vi "inclino._up3.vi"() -> ()   [LabVIEW 2023]
doc: "This example performs a serial port write and a serial port read. The parameters set for the serial port must match the parameters of the connected instrument or device. The VISA Configure Serial Port VI sets the configuration parameters. The front panel displays the controls used to configure the basic parameters, such as baud rate, data bits, and parity. The VI passes the VISA resource name to other VIs that perform operations on that VISA resource. The VISA Write function sends a command to the serial device and the VISA Read function returns data based on the command. The VISA Close function then closes the reference to the serial device. It is important to close the reference; otherwise, further communication through that port might not be possible."
uses:
  <vilib>/Instr/_visa.llb/VISA Configure Serial Port (Instr).vi
  Program Files (x86)/National Instruments/LabVIEW 2023/examples/Instrument IO/Serial/support/Serial - Settings.ctl
panel:
  out "Connected":bool
  out "Error Status":bool
  out "Connected":bool
  out "Error status":bool
  in  "Tab Control":enum32{"Page 1", "Page 2"}(tab)
  out "XY Graph":cluster{dbl[], dbl[]}(graph)
  out "VISA resource name out 2":refnum<visa-resource-name>
  out "VISA resource name out":refnum<visa-resource-name>
  out "?":dbl[][](array[numeric])
  in  "Referance Angle":string="!157:SOUT?\n"
  in  "Angle":string="!157:SOUT?\n"
  in  "Stop":bool
  out "?":dbl(knob) scale=-60.0..60.0
  out "?":dbl(knob) scale=-60.0..60.0
  out "Angle":dbl
  in  "Serial Settings 2":T1={"baud rate"=9600, "data bits"=8, "parity"=enum."None", "stop bits"=10, "flow control"=0} {"flow control" items=["None"=0, "XON/XOFF"=1, "RTS/CTS"=2, "DTR/DSR"=4]; "stop bits" items=["1.0"=10, "1.5"=15, "2.0"=20]; "data bits" min=5 max=8 step=1; "baud rate" items=["75"=75, "110"=110, "134"=134, "150"=150, "300"=300, "600"=600, "1200"=1200, "1800"=1800, "2400"=2400, "4800"=4800, "7200"=7200, "9600"=9600, "14400"=14400, "19200"=19200, "28800"=28800, "38400"=38400, "56000"=56000, "57600"=57600, "115200"=115200, "128000"=128000, "230400"=230400]}
  in  "PORT":refnum<visa-resource-name>="COM1"
  out "error out 2":errorcluster
  out "error out":errorcluster
  out "Referance  Angle":dbl
  in  "Serial Settings":T1={"baud rate"=9600, "data bits"=8, "parity"=enum."None", "stop bits"=10, "flow control"=0} {"flow control" items=["None"=0, "XON/XOFF"=1, "RTS/CTS"=2, "DTR/DSR"=4]; "stop bits" items=["1.0"=10, "1.5"=15, "2.0"=20]; "data bits" min=5 max=8 step=1; "baud rate" items=["75"=75, "110"=110, "134"=134, "150"=150, "300"=300, "600"=600, "1200"=1200, "1800"=1800, "2400"=2400, "4800"=4800, "7200"=7200, "9600"=9600, "14400"=14400, "19200"=19200, "28800"=28800, "38400"=38400, "56000"=56000, "57600"=57600, "115200"=115200, "128000"=128000, "230400"=230400]}
  in  "PORT":refnum<visa-resource-name>="COM1"
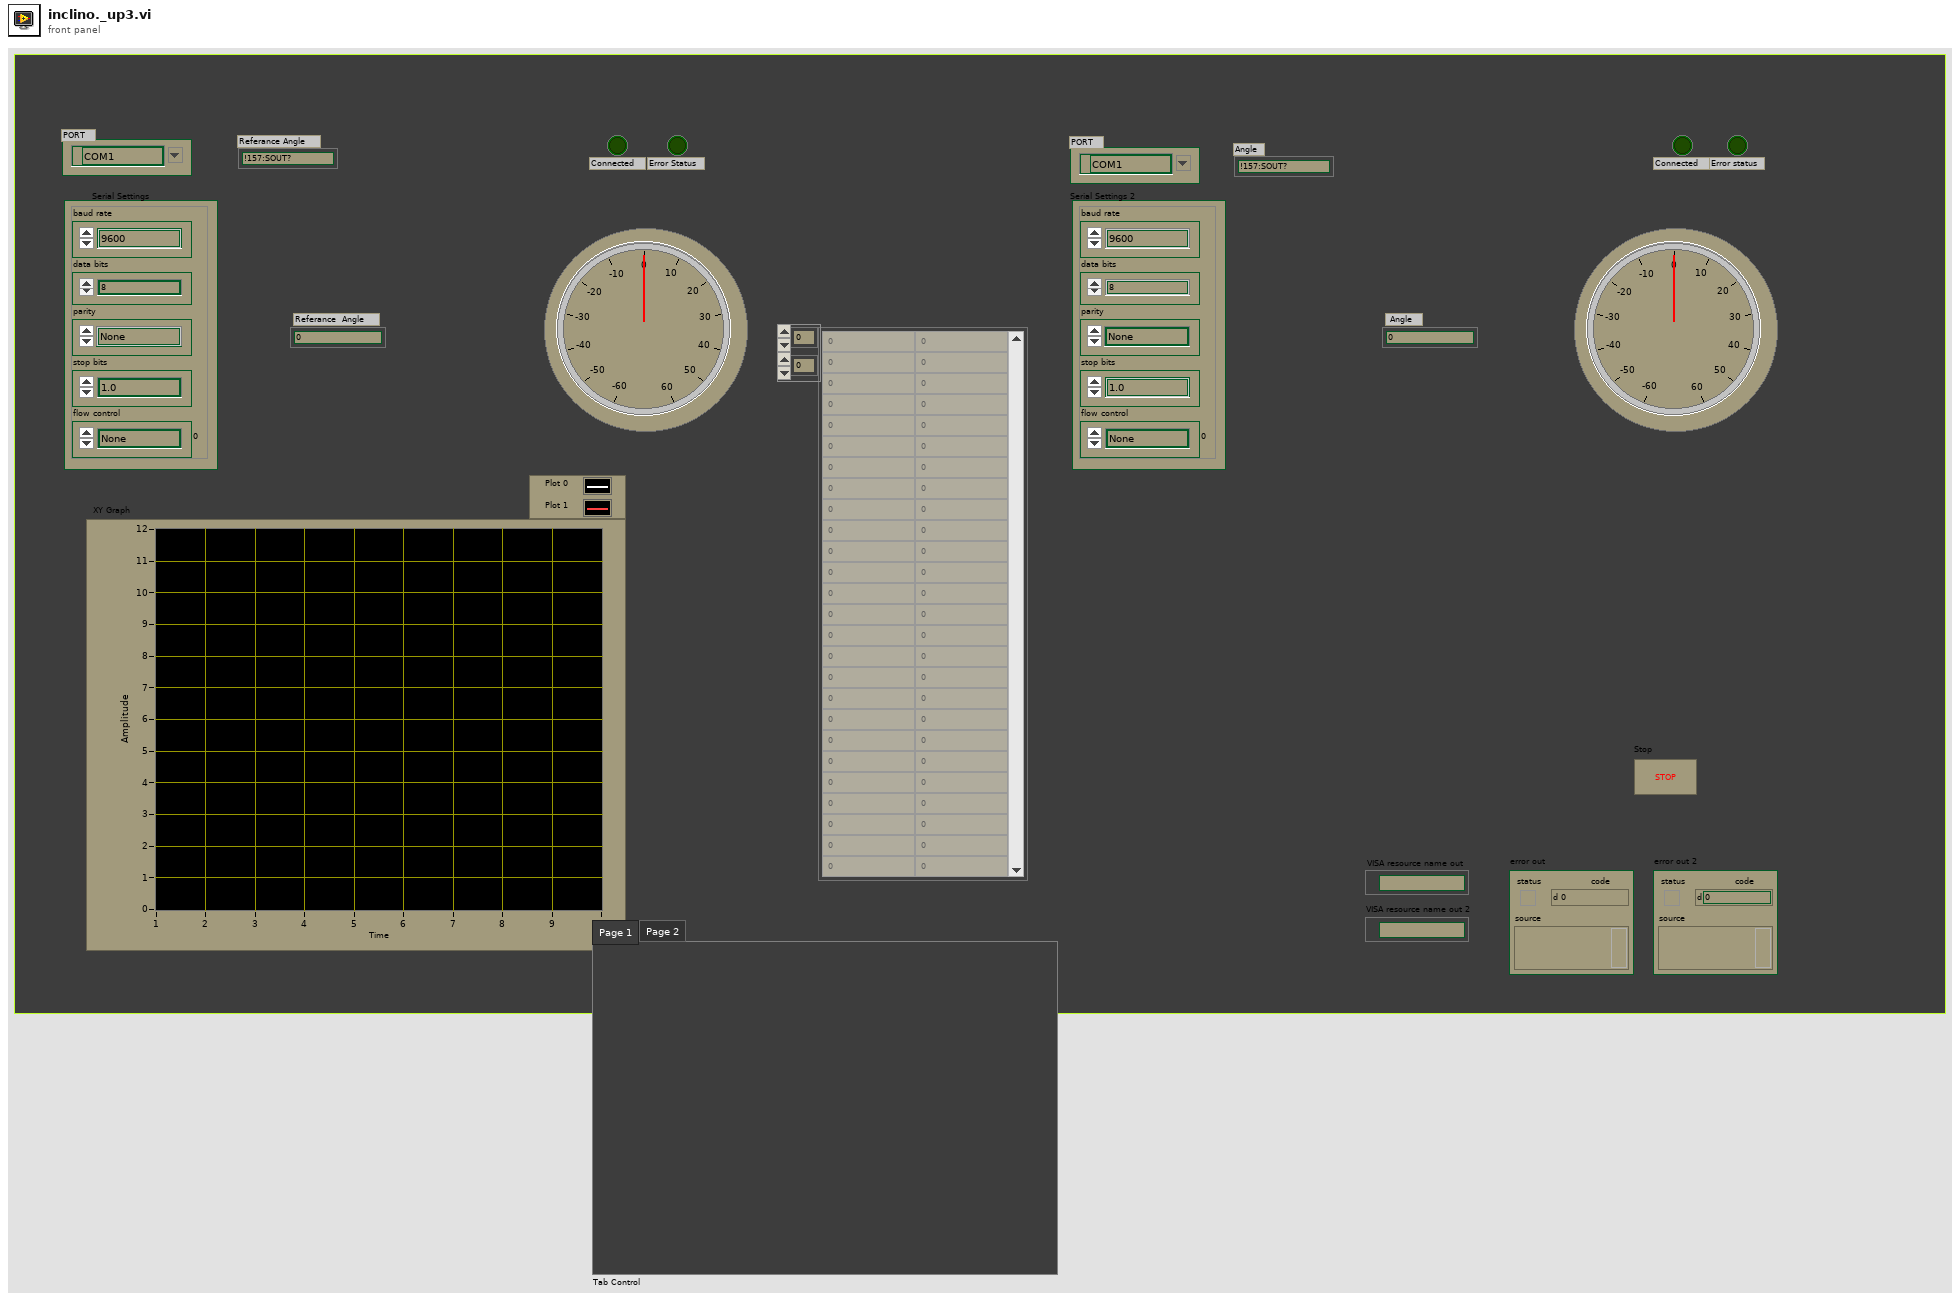
[diagram p1: front panel]
types:
  T1 = typedef "Serial - Settings.ctl" = cluster{"baud rate":u32, "data bits":u16, "parity":enum16{"None", "Odd", "Even", "Mark", "Space"}, "stop bits":u16, "flow control":u16}
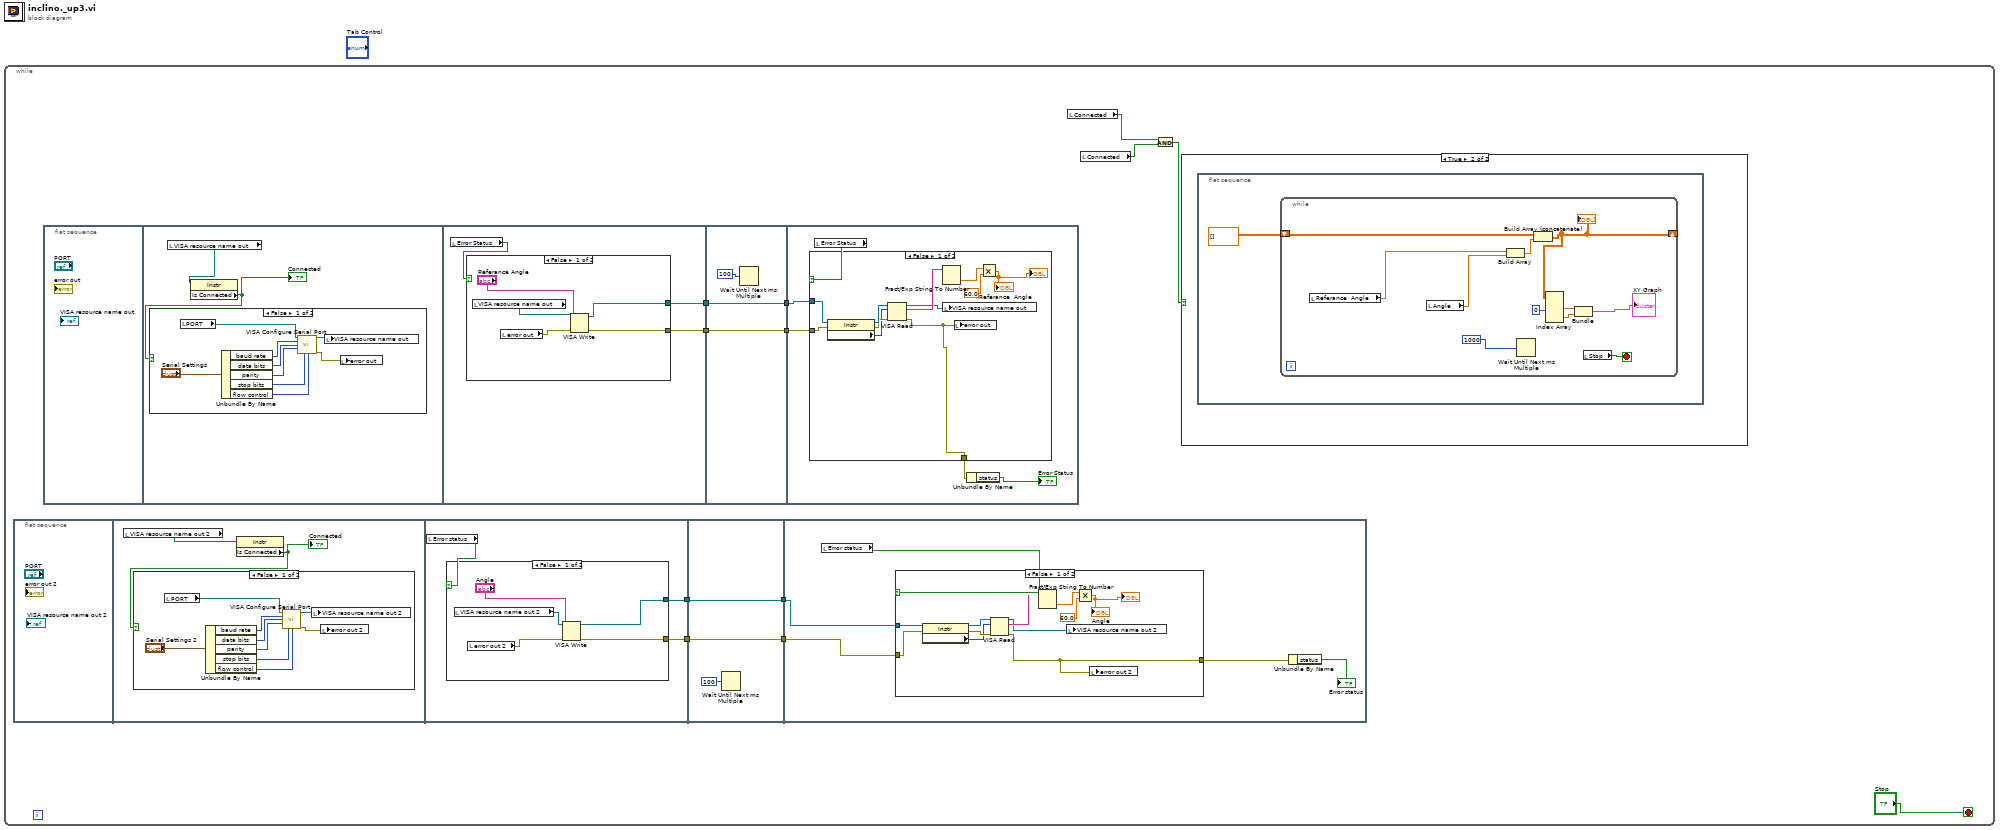
[diagram p0: block diagram]
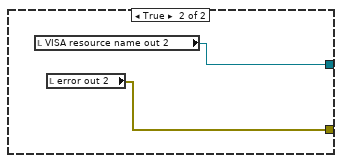
[diagram p4: hidden frame]
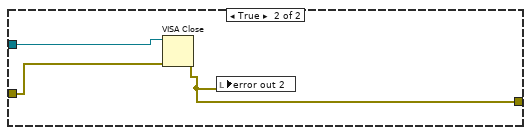
[diagram p5: hidden frame]
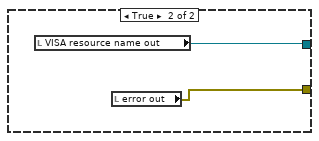
[diagram p7: hidden frame]
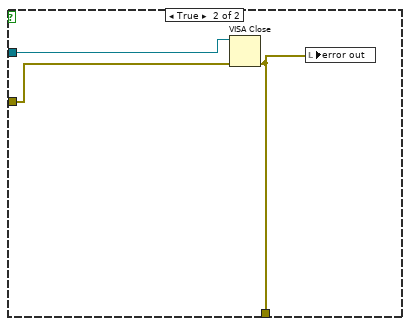
[diagram p8: hidden frame]
diagram:
  n1 = while {
    stop <- "Stop" stop-if-true
    n2 = flat-sequence {
      tunnel: [w38] -> w6
      tunnel: [w37] -> w4
      tunnel: [w47] -> w7
      tunnel: w6 -> [w47]
      tunnel: [w46] -> w5
      tunnel: w4 -> [w46]
      tunnel: w5 -> [w50]
      tunnel: w7 -> [w51]
      frame #0 {
      }
      frame #1 {
        n3 = local read "VISA resource name out 2"() -> (w26:refnum<visa-resource-name>)
        n4 = property class="Instr"(reference=w26) -> ("Is Connected"=w25:bool)  [unwired: 1 in, 2 out]
        "Connected" <- w25
        n5 = case shown="False" w25 {
          frame False {
            n6 = local read "PORT"() -> (w29:refnum<visa-resource-name>)
            n7 = Unbundle By Name("Serial Settings 2") -> ("baud rate"=w30:u32, "data bits"=w31:u16, "parity"=w32:enum16{"None", "Odd", "Even", "Mark", "Space"}, "stop bits"=w33:u16, "flow control"=w34:u16)
            n8 = call-poly "VISA Configure Serial Port"("VISA resource name"=w29, "baud rate (9600)"=w30, "data bits (8)"=w31, "parity (0:none)"=w32, "stop bits (10: 1 bit)"=w33, "flow control (0:none)"=w34) -> ("VISA resource name out"=w28:refnum<visa-resource-name>, "error out"=w27:errorcluster)  [unwired: 3 in, 5 out]
            n9 = local write "VISA resource name out 2"(w28) -> ()
            n10 = local write "error out 2"(w27) -> ()
          }
          frame True {
          }
        }
      }
      frame #2 {
        n11 = local read "Error status"() -> (w36:bool)
        n12 = case shown="False" w36 {
          tunnel: [w42 w45] -> w38
          tunnel: [w41 w44] -> w37
          frame False {
            n13 = local read "VISA resource name out 2"() -> (w39:refnum<visa-resource-name>)
            n14 = local read "error out 2"() -> (w40:errorcluster)
            n15 = VISA Write(VISA resource name=w39, write buffer="Angle", error in (no error)=w40) -> (VISA resource name out=w42:refnum<visa-resource-name>, error out=w41:errorcluster)  [unwired: 1 out]
          }
          frame True {
            n16 = local read "VISA resource name out 2"() -> (w45:refnum<visa-resource-name>)
            n17 = local read "error out 2"() -> (w44:errorcluster)
          }
        }
      }
      frame #3 {
        n18 = Wait Until Next ms Multiple(millisecond multiple=u32 100) -> ()  [unwired: 1 out]
      }
      frame #4 {
        n19 = local read "Error status"() -> (w53:bool)
        n20 = case shown="False" w53 {
          tunnel: w51 -> [w60 w67]
          tunnel: w50 -> [w59 w66]
          tunnel: [w55 w65] -> w49
          frame False {
            n21 = property class="Instr"(reference=w60, error in=w59) -> (reference out=w58:refnum<visa-resource-name>, error out=w57:errorcluster, "Serial Settings:Number of Bytes at Serial Port"=w56:u32)
            n22 = VISA Read(VISA resource name=w58, byte count=w56, error in (no error)=w57) -> (VISA resource name out=w54:refnum<visa-resource-name>, read buffer=w61:string, error out=w55:errorcluster)  [unwired: 1 out]
            n23 = Fract/Exp String To Number(string=w61) -> (number=w64:dbl)  [unwired: 3 in, 1 out]
            n24 = local write "VISA resource name out 2"(w54) -> ()
            n25 = Multiply(x=w64, y=60.0) -> (x*y=→"Angle" →"?":dbl)
            n26 = local write "error out 2"(w55) -> ()
          }
          frame True {
            n27 = VISA Close(VISA resource name=w67, error in (no error)=w66) -> (error out=w65:errorcluster)
            n28 = local write "error out 2"(w65) -> ()
          }
        }
        n29 = Unbundle By Name(w49) -> ("status"=→"Error status":bool)
      }
    }
    n30 = flat-sequence {
      tunnel: [w81] -> w10
      tunnel: [w80] -> w8
      tunnel: [w90] -> w11
      tunnel: w10 -> [w90]
      tunnel: [w89] -> w9
      tunnel: w8 -> [w89]
      tunnel: w9 -> [w93]
      tunnel: w11 -> [w94]
      frame #0 {
      }
      frame #1 {
        n31 = local read "VISA resource name out"() -> (w69:refnum<visa-resource-name>)
        n32 = property class="Instr"(reference=w69) -> ("Is Connected"=w68:bool)  [unwired: 1 in, 2 out]
        "Connected" <- w68
        n33 = case shown="False" w68 {
          frame False {
            n34 = local read "PORT"() -> (w72:refnum<visa-resource-name>)
            n35 = Unbundle By Name("Serial Settings") -> ("baud rate"=w73:u32, "data bits"=w74:u16, "parity"=w75:enum16{"None", "Odd", "Even", "Mark", "Space"}, "stop bits"=w76:u16, "flow control"=w77:u16)
            n36 = call-poly "VISA Configure Serial Port"("VISA resource name"=w72, "baud rate (9600)"=w73, "data bits (8)"=w74, "parity (0:none)"=w75, "stop bits (10: 1 bit)"=w76, "flow control (0:none)"=w77) -> ("VISA resource name out"=w71:refnum<visa-resource-name>, "error out"=w70:errorcluster)  [unwired: 3 in, 5 out]
            n37 = local write "VISA resource name out"(w71) -> ()
            n38 = local write "error out"(w70) -> ()
          }
          frame True {
          }
        }
      }
      frame #2 {
        n39 = local read "Error Status"() -> (w79:bool)
        n40 = case shown="False" w79 {
          tunnel: [w85 w88] -> w81
          tunnel: [w84 w87] -> w80
          frame False {
            n41 = local read "VISA resource name out"() -> (w82:refnum<visa-resource-name>)
            n42 = local read "error out"() -> (w83:errorcluster)
            n43 = VISA Write(VISA resource name=w82, write buffer="Referance Angle", error in (no error)=w83) -> (VISA resource name out=w85:refnum<visa-resource-name>, error out=w84:errorcluster)  [unwired: 1 out]
          }
          frame True {
            n44 = local read "VISA resource name out"() -> (w88:refnum<visa-resource-name>)
            n45 = local read "error out"() -> (w87:errorcluster)
          }
        }
      }
      frame #3 {
        n46 = Wait Until Next ms Multiple(millisecond multiple=u32 100) -> ()  [unwired: 1 out]
      }
      frame #4 {
        n47 = local read "Error Status"() -> (w95:bool)
        n48 = case shown="False" w95 {
          tunnel: w94 -> [w103 w110]
          tunnel: w93 -> [w102 w109]
          tunnel: [w97 w108] -> w92
          frame False {
            n49 = property class="Instr"(reference=w103, error in=w102) -> (reference out=w101:refnum<visa-resource-name>, error out=w100:errorcluster, "Serial Settings:Number of Bytes at Serial Port"=w99:u32)
            n50 = VISA Read(VISA resource name=w101, byte count=w99, error in (no error)=w100) -> (VISA resource name out=w98:refnum<visa-resource-name>, read buffer=w105:string, error out=w97:errorcluster)  [unwired: 1 out]
            n51 = Fract/Exp String To Number(string=w105) -> (number=w107:dbl)  [unwired: 3 in, 1 out]
            n52 = local write "VISA resource name out"(w98) -> ()
            n53 = local write "error out"(w97) -> ()
            n54 = Multiply(x=w107, y=60.0) -> (x*y=→"Referance  Angle" →"?":dbl)
          }
          frame True {
            n55 = VISA Close(VISA resource name=w110, error in (no error)=w109) -> (error out=w108:errorcluster)
            n56 = local write "error out"(w108) -> ()
          }
        }
        n57 = Unbundle By Name(w92) -> ("status"=→"Error Status":bool)
      }
    }
    n58 = local read "Connected"() -> (w3:bool)
    n59 = local read "Connected"() -> (w2:bool)
    n60 = And(x=w3, y=w2) -> (x .and. y?=w1:bool)
    n61 = case shown="True" w1 {
      frame False {
      }
      frame True {
        n62 = flat-sequence {
          frame #0 {
            n63 = while {
              shift-right: [w19] -> _
              shift-left: dbl[][] [] -> [w23]
              stop <- w14 stop-if-true
              n64 = local read "Referance  Angle"() -> (w20:dbl)
              n65 = local read "Angle"() -> (w21:dbl)
              n66 = Build Array(w20, w21) -> (w24:dbl[])
              n67 = Wait Until Next ms Multiple(millisecond multiple=u32 1000 ("milliseconds to wait")) -> ()  [unwired: 1 out]
              n68 = Build Array (concatenate)(w23, w24) -> (w19:dbl[][])
              "?" <- w19
              n69 = Index Array(array=w19, index (col) #1=0 ("disabled index (col)")) -> (element #1=w17:dbl[], element #2=w16:dbl[])  [unwired: 3 in]
              n70 = Bundle(w17, w16) -> (→"XY Graph":cluster{dbl[], dbl[]})  [unwired: 1 in]
              n71 = local read "Stop"() -> (w14:bool)
            }
          }
        }
      }
    }
  }
